vi "Ignore-error-single.vi"(8 "error in (no error)":errorcluster, 10 "Error to ignore (1)":i32=1) -> (0 "error out":errorcluster)   [LabVIEW 2013, in "SLMControl.lvlib" / "SC-Main.lvclass"]
uses:
  SC-Main.lvclass
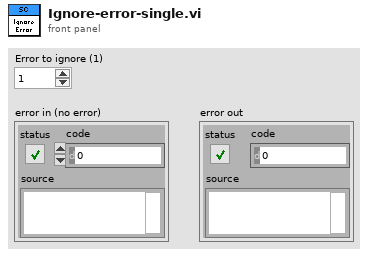
[diagram p1: front panel]
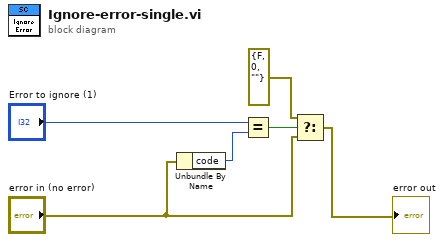
[diagram p0: block diagram]
diagram:
  n1 = Unbundle By Name("error in (no error)") -> ("code"=w2:i32)
  n2 = Equal?(x="Error to ignore (1)", y=w2) -> (x = y?=w3:bool)
  n3 = Select(t=errorcluster {"status"=FALSE, "code"=0, "source"=""} ("error constant"), s=w3, f="error in (no error)") -> (s? t:f=→"error out":errorcluster)
